vi "Arrange Vertical.vi"(8 "error in (no error)":errorcluster, 11 "[MDI] Parent in":refnum<class "[MDI] Parent.lvclass">) -> (0 "error out":errorcluster, 3 "[MDI] Parent out":refnum<class "[MDI] Parent.lvclass">)   [LabVIEW 2020, in "[MDI] Parent.lvlib" / "[MDI] Parent.lvclass"]
uses:
  [MDI] Parent.lvclass
  [MDI] Parent.lvclass/[MDI] Parent.ctl
  user32.dll
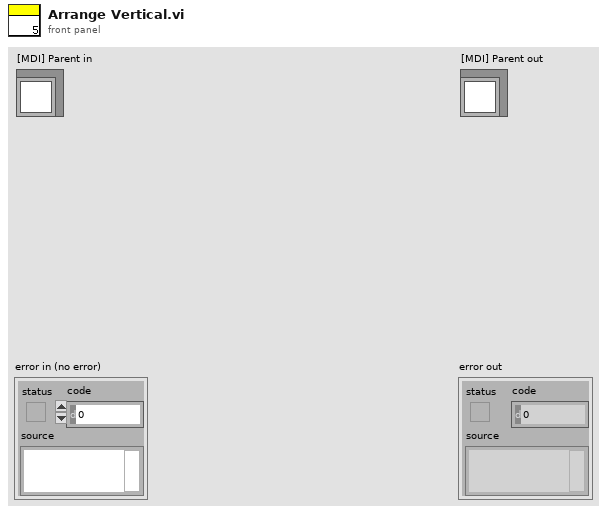
[diagram p1: front panel]
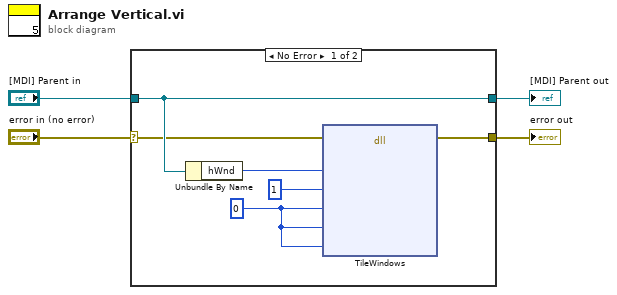
[diagram p0: block diagram]
diagram:
  n1 = case shown="No Error" "error in (no error)" {
    selector: "error in (no error)" -> [w9 w12]
    tunnel: [w8 w12] -> w3
    tunnel: [w10 w11] -> w1
    tunnel: "[MDI] Parent in" -> [w10 w11]
    frame No Error {
      w7 = u32 0 ("wHow")
      n2 = Unbundle By Name(w10) -> ("hWnd"=w6:u32)
      n3 = dll-call lib="user32.dll" fn="TileWindows"(error in=w9, "hWndParent"=w6, "wHow"=u32 1, "rect"=w7, "cKids"=w7, "IpKids"=w7) -> (error out=w8:errorcluster)  [unwired: 8 in, 1 out]
    }
    frame Error {
    }
  }
  "error out" <- w3
  "[MDI] Parent out" <- w1
